vi "IntersectLinesDegen.vi"(10 "Line2D_2":T2, 11 "Line2D_1":T2) -> (2 "Intersect?":bool, 3 "Intersection1":T1)   [LabVIEW 2014]
uses:
  TypeDefs/Line2DnoSlope.ctl
  TypeDefs/Point2D.ctl
panel:
  out "NumberOfIntersections":i32
  out "Intersection2":T1
  out "Denom":dbl
  out "Num":dbl
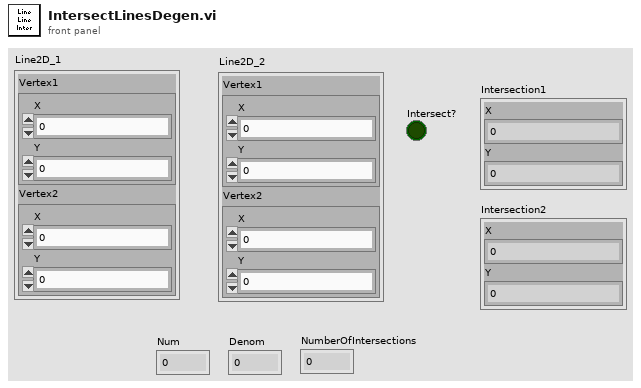
[diagram p1: front panel]
types:
  T1 = typedef "Point2D.ctl" = cluster{"X":sgl, "Y":sgl}
  T2 = typedef "Line2DnoSlope.ctl" = cluster{"Vertex1":T1, "Vertex2":T1}
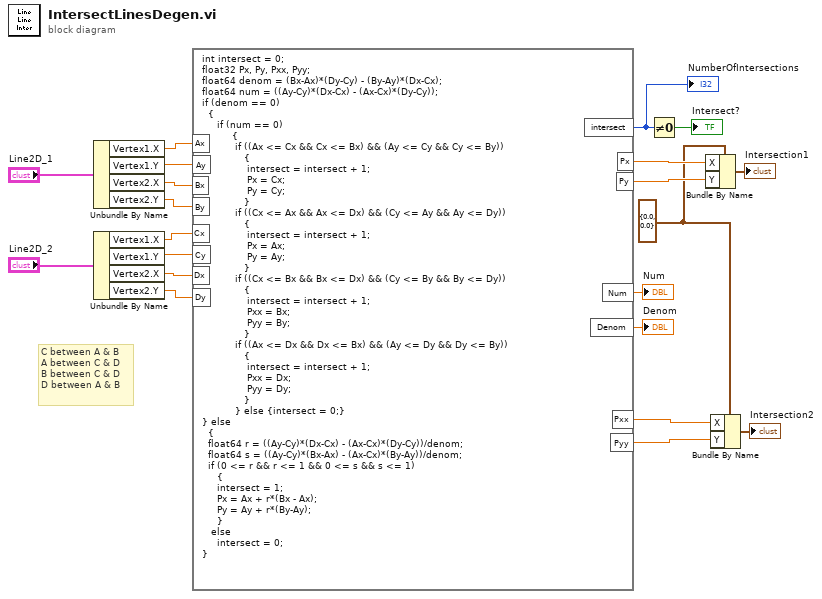
[diagram p0: block diagram]
diagram:
  w3 = T1 {"X"=0.0, "Y"=0.0} ("Point2D")
  # "C between A & B\nA between C & D\nB between C & D\nD between A & B"
  n1 = Unbundle By Name("Line2D_1") -> ("Vertex1.X"=w19:sgl, "Vertex1.Y"=w18:sgl, "Vertex2.X"=w17:sgl, "Vertex2.Y"=w16:sgl)
  n2 = Unbundle By Name("Line2D_2") -> ("Vertex1.X"=w15:sgl, "Vertex1.Y"=w14:sgl, "Vertex2.X"=w13:sgl, "Vertex2.Y"=w12:sgl)
  n3 = formula code="int intersect = 0;\nfloat32 Px, Py, Pxx, Pyy;\nfloat64 denom = (Bx-Ax)*(Dy-Cy) - (By-Ay)*(Dx-Cx);\nfloat64 num = ((Ay-Cy)*(Dx-Cx) - (Ax-Cx)*(Dy-Cy));\nif (denom == 0)\n  {\n     if (num == 0) \n          {\n           if ((Ax <= Cx && Cx <= Bx) && (Ay <= Cy && Cy <= By))\n              {\n               intersect = intersect + 1;\n               Px = Cx;\n               Py = Cy;\n              }\n           if ((Cx <= Ax && Ax <= Dx) && (Cy <= Ay && Ay <= Dy))\n              {\n               intersect = intersect + 1;\n               Px = Ax;\n               Py = Ay;\n              }\n           if ((Cx <= Bx && Bx <= Dx) && (Cy <= By && By <= Dy))\n              {\n               intersect = intersect + 1;\n               Pxx = Bx;\n               Pyy = By;\n              }\n           if ((Ax <= Dx && Dx <= Bx) && (Ay <= Dy && Dy <= By))\n              {\n               intersect = intersect + 1;\n               Pxx = Dx;\n               Pyy = Dy;\n              }\n           } else {intersect = 0;}\n} else\n  {\n  float64 r = ((Ay-Cy)*(Dx-Cx) - (Ax-Cx)*(Dy-Cy))/denom;\n  float64 s = ((Ay-Cy)*(Bx-Ax) - (Ax-Cx)*(By-Ay))/denom;\n  if (0 <= r && r <= 1 && 0 <= s && s <= 1)\n     {\n     intersect = 1;\n     Px = Ax + r*(Bx - Ax);\n     Py = Ay + r*(By-Ay);\n     }\n   else\n     intersect = 0;\n}"("Ax"=w19, "Ay"=w18, "Bx"=w17, "By"=w16, "Cx"=w15, "Cy"=w14, "Dx"=w13, "Dy"=w12) -> ("intersect"=w11:i32, "Px"=w9:sgl, "Py"=w8:sgl, "Num"=→"Num":dbl, "Denom"=→"Denom":dbl, "Pxx"=w2:sgl, "Pyy"=w1:sgl)
  "NumberOfIntersections" <- w11
  n4 = Not Equal To 0?(x=w11) -> (x != 0?=→"Intersect?":bool)
  n5 = Bundle By Name(cluster=w3, "X"=w9, "Y"=w8) -> (→"Intersection1":T1)
  n6 = Bundle By Name(cluster=w3, "X"=w2, "Y"=w1) -> (→"Intersection2":T1)
